vi "Math - Offset Signals.vi"(0 "reference in":refnum<class "GSwFormDSP.lvclass">, 5 "error in (no error)":errorcluster, 6 "Anotate Signal Name":bool=TRUE, 7 "Offsets":dbl[](array[numeric])=[0.0]) -> (14 "reference in":refnum<class "GSwFormDSP.lvclass">, 19 "error out":errorcluster)   [LabVIEW 2022 SP3, in "GSwFormDSP.lvclass"]
uses:
  GSwFormDSP.lvclass
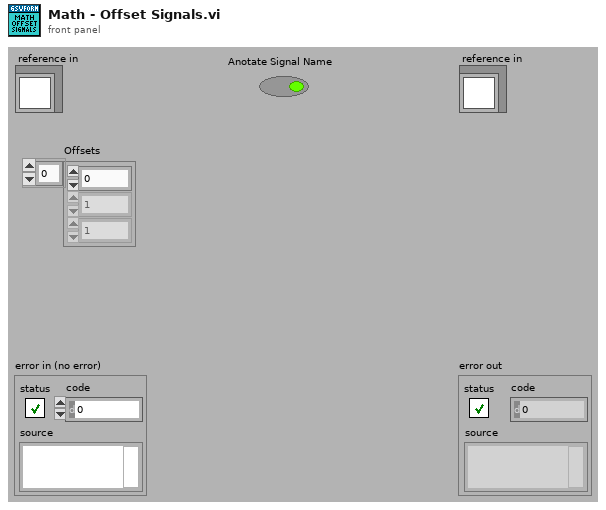
[diagram p1: front panel]
types:
  T1 = typedef "GSwFormDSP.lvclass/ObjectAttributesRef.ctl" = refnum<data-value>
  T2 = typedef "GSwFormDSP.lvclass/ObjectAttributes.ctl" = cluster{"Wform Ref":refnum<data-value>, "Nb Signals":i32, "Spectral Function Parameters":T3, "FFT":waveform(cdb)[], "Nb FFT":i32, "Nb Averages":i32[], "Reference Indexes":i32[], "Response Indexes":i32[], "Coherence":waveform(dbl)[], "TDF Parameters":T5, "DAQ":cluster{"Duration (sec)":dbl, "Buffer Size (Samples)":i32, "Offset (Samples)":i32}, "Filter Impulse Response (TDF)":waveform(dbl), "Sound Playback":T6}
  T3 = typedef "GSwFormDSP.lvclass/Spectral Parameters.ctl" = cluster{"Frequency resolution (Hz)":dbl, "Overlap":dbl, "Window":T4}
  T4 = typedef "NI_AALPro.lvlib/windowTd.ctl" = u32
  T5 = typedef "GSwFormDSP.lvclass/TDF Parameters.ctl" = cluster{"Filter":enum32{"Lowpass", "Highpass", "Bandpass", "Bandstop"}, "Type:":enum16{"Butterworth", "Chebyshev", "Inv Chebyshev", "Elliptic", "Bessel"}, "LP cutoff freq":dbl, "HP cutoff freq":dbl, "Order":i32, "passband ripple (dB)":dbl, "stopband attenuation (dB)":dbl, "Phaseless Filter":bool, "Include Fade IN and OUT":bool}
  T6 = typedef "GSwFormDSP.lvclass/Sound Playback.ctl" = cluster{"Timer start (ms)":u32, "task ID":T7, "Cursor Init Location (s)":dbl, "SC Volume":dbl}
  T7 = typedef "Sound Output Task ID.ctl" = u32
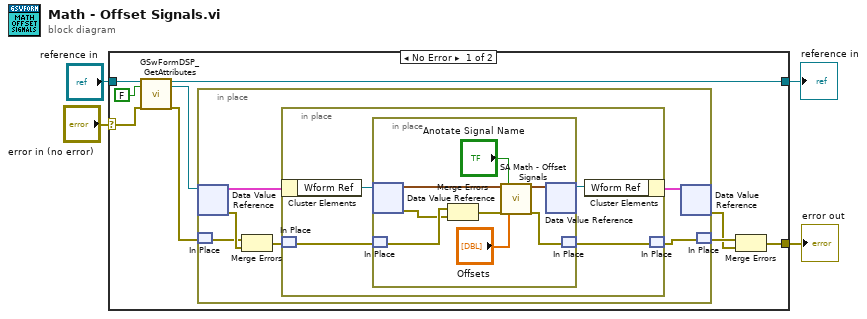
[diagram p0: block diagram]
diagram:
  n1 = case shown="No Error" "error in (no error)" {
    selector: "error in (no error)" -> [w10 w33]
    tunnel: [w13 w33] -> w3
    tunnel: [w8 w32] -> w1
    tunnel: "reference in" -> [w11 w32]
    frame No Error {
      n2 = call "GSwFormDSP_GetAttributes.vi"("reference in"=w11, "return data? (T)"=FALSE, "error in (no error)"=w10) -> ("reference out"=w8:refnum<class "GSwFormDSP.lvclass">, "attributes ref"=w9:T1, "error out"=w7:errorcluster)  [unwired: 13 in, 1 out]
      n3 = in-place {
        n4 = in-place-dvr #1(w9) -> (w17:T2, w19:errorcluster)
        n5 = in-place-match #2(w7) -> (w18:errorcluster)
        n6 = Merge Errors(w18, w19) -> (w16:errorcluster)
        n7 = in-place {
          n8 = in-place-cluster #3(w17) -> ("Wform Ref"=w23:refnum<data-value>)
          n9 = in-place-match #4(w16) -> (w21:errorcluster)
          n10 = in-place {
            n11 = in-place-dvr #5(w23) -> (w30:waveform(dbl)[], w24:errorcluster)
            n12 = in-place-match #6(w21) -> (w26:errorcluster)
            n13 = Merge Errors(w26, w24) -> (w25:errorcluster)
            n14 = call "SA Math - Offset Signals.vi"("Signal IN"=w30, "error in (no error)"=w25, "Anotate Signal Name"="Anotate Signal Name", "Offset Values"="Offsets") -> ("Signal OUT"=w31:waveform(dbl)[], "error out"=w27:errorcluster)  [unwired: 14 in]
            n15 = in-place-dvr #5(w31) -> (w22:refnum<data-value>)  [unwired: 1 out]
            n16 = in-place-match #6(w27) -> (w20:errorcluster)
          }
          n17 = in-place-cluster #3("Wform Ref"=w22) -> (w15:T2)
          n18 = in-place-match #4(w20) -> (w14:errorcluster)
        }
        n19 = in-place-dvr #1(w15) -> (w5:errorcluster)  [unwired: 1 out]
        n20 = in-place-match #2(w14) -> (w6:errorcluster)
      }
      n21 = Merge Errors(w6, w5) -> (w13:errorcluster)
    }
    frame Error {
    }
  }
  "error out" <- w3
  "reference in" <- w1
